vi "open.vi"(8 "error in":errorcluster, 11 "IP Address (LJM_idANY )":string="LJM_idANY ") -> (0 "error out":errorcluster, 2 "Connection Info":T1, 3 "Handle":i32)   [LabVIEW 2025, in "LabJackEKG.lvlib"]
uses:
  LabJackEKG.lvlib
  Typedefs/ConnectionInfo.ctl
panel:
  # "LabJack V0.10\nOpen"
  # "09.05.2025"
  # "Blaz Kelbl"
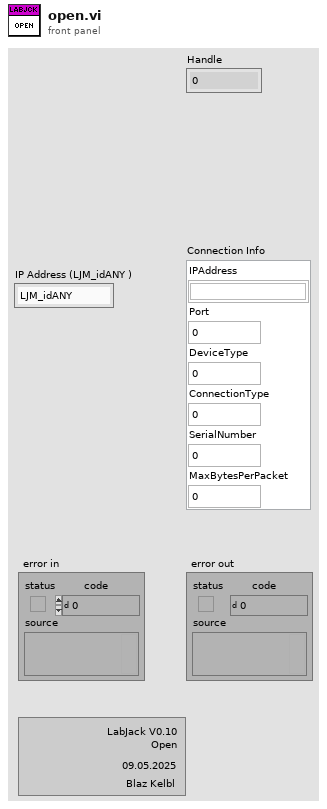
[diagram p1: front panel]
types:
  T1 = typedef "LabJackEKG.lvlib/ConnectionInfo.ctl" = cluster{"IPAddress":string, "Port":i32, "DeviceType":i32, "ConnectionType":i32, "SerialNumber":i32, "MaxBytesPerPacket":i32}
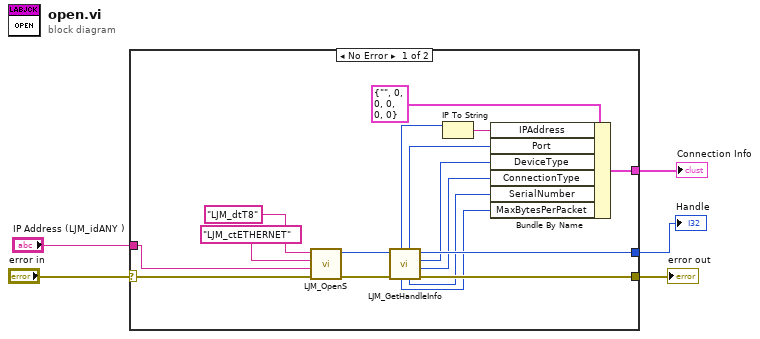
[diagram p0: block diagram]
diagram:
  n1 = case shown="No Error" "error in" {
    selector: "error in" -> [w22 w23]
    tunnel: [w18 w23] -> w4
    tunnel: [w20 _] -> w3
    tunnel: [w16 _] -> w2
    tunnel: "IP Address (LJM_idANY )" -> [w6 _]
    frame No Error {
      n2 = call <vilib>:"LJM_OpenS.vi"("error in"=w22, "Identifier"=w6, "ConnectionType"="LJM_ctETHERNET", "DeviceType"="LJM_dtT8") -> ("error out"=w19:errorcluster, "Handle"=w17:i32)  [unwired: 6 in]
      n3 = call <vilib>:"LJM_GetHandleInfo.vi"("error in"=w19, "Handle In"=w17) -> ("error out"=w18:errorcluster, "ConnectionType"=w12:i32, "DeviceType"=w13:i32, "Handle Out"=w16:i32, "SerialNumber"=w11:i32, "Port"=w14:i32, "MaxBytesPerPacket"=w10:i32, "IPAddress"=w15:i32)  [unwired: 2 in]
      n4 = IP To String(2:w15) -> (0:w9:string)  [unwired: 1 in]
      n5 = Bundle By Name(cluster=T1 {"IPAddress"="", "Port"=0, "DeviceType"=0, "ConnectionType"=0, "SerialNumber"=0, "MaxBytesPerPacket"=0} ("Cluster"), "IPAddress"=w9, "Port"=w14, "DeviceType"=w13, "ConnectionType"=w12, "SerialNumber"=w11, "MaxBytesPerPacket"=w10) -> (w20:T1)
    }
    frame Error {
    }
  }
  "error out" <- w4
  "Handle" <- w2
  "Connection Info" <- w3
